vi "File.Folder, Move or Copy.vi"(8 "error in (no error)":errorcluster, 9 "Action":enum16{"Move", "Copy"}(ring), 10 "Dest":path, 11 "Source":path) -> (0 "error out":errorcluster, 3 "Dest Dup":path)   [LabVIEW 2024]
uses:
  Errors/Error.Error Code List.ctl
  <vilib>/KATE/Files/File Utils.lvlib
  Errors.lvlib
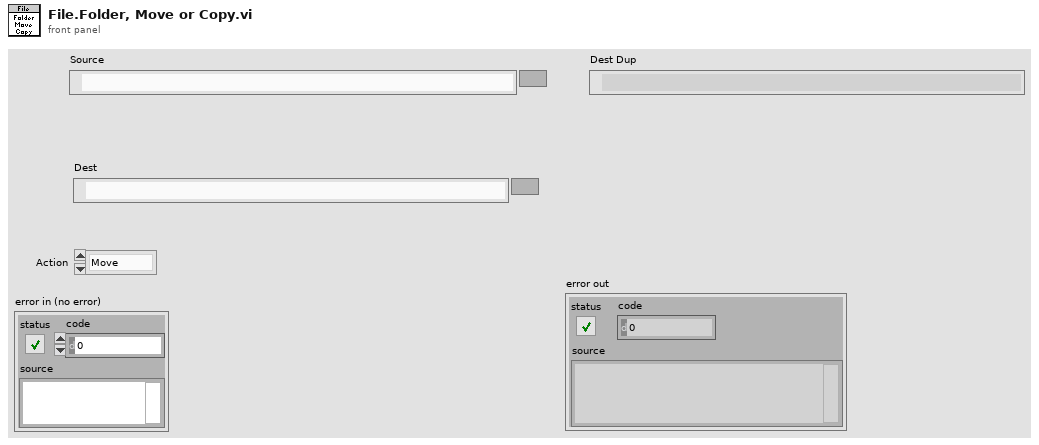
[diagram p1: front panel]
types:
  T1 = typedef "EQMF.lvlib/Errors.lvlib/Error.Error Code List.ctl" = i32
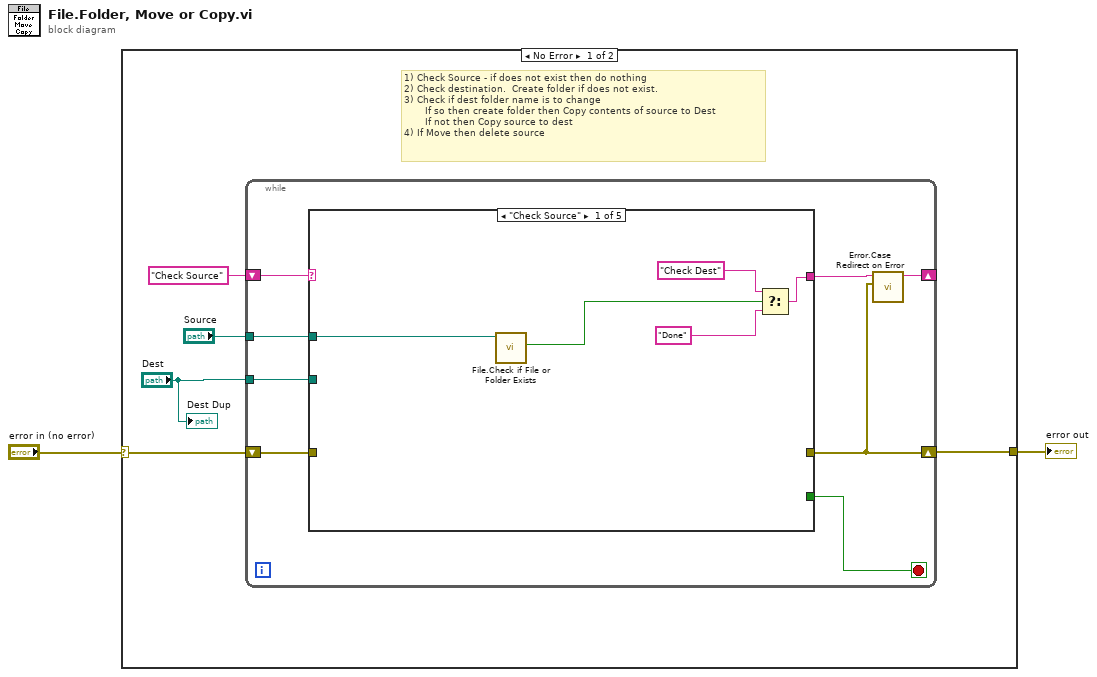
[diagram p0: block diagram]
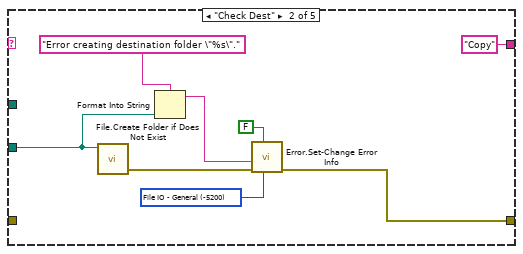
[diagram p2: hidden frame]
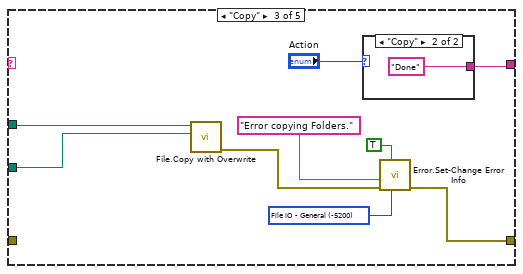
[diagram p3: hidden frame]
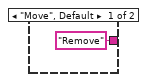
[diagram p4: hidden frame]
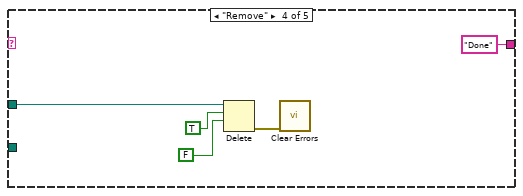
[diagram p5: hidden frame]
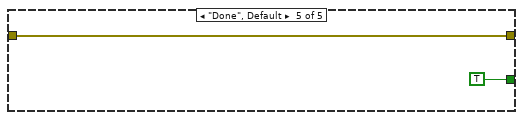
[diagram p6: hidden frame]
diagram:
  n1 = case shown="No Error" "error in (no error)" {
    selector: "error in (no error)" -> [w5 w47]
    tunnel: [w3 w47] -> w1
    frame No Error {
      # "1) Check Source - if does not exist then do nothing\n2) Check destination.  Create folder if does not exist.\n3) Check if dest folder name is to change\n       If so then create folder then Copy contents of source to Dest\n       If not then Copy source to dest\n4) If Move then delete source"
      n2 = while {
        shift-right: [w14] -> _
        shift-left: "Check Source" -> [w15]
        tunnel: "Source" -> [w12]
        tunnel: "Dest" -> [w11]
        shift-right: [w9] -> w3
        shift-left: w5 -> [w10]
        stop <- w8 stop-if-true
        n3 = case shown="\"Check Source\"" w15 {
          tunnel: [w19 "Copy" w36 "Done" _] -> w13
          tunnel: w12 -> [w17 _ w35 w43 _]
          tunnel: w11 -> [_ w25 w34 _ _]
          tunnel: w10 -> [_ _ _ _ w46]
          tunnel: [_ w22 w29 _ w46] -> w9
          tunnel: [_ _ _ _ TRUE] -> w8
          frame "Check Source" {
            n4 = call <vilib>:"File.Check if File or Folder Exists.vi"("Path"=w17) -> ("Exists"=w16:bool)  [unwired: 6 in, 4 out]
            n5 = Select(t="Check Dest", s=w16, f="Done") -> (s? t:f=w19:string)
          }
          frame "Check Dest" {
            w23 = T1 -5200 items=["No Error"=0, "Abort"=-2, "Misc"=-5000, "Fixture Error"=-5100, "File IO - General"=-5200, "FIle IO - Config Error"=-5201, "Instrument - General"=-5300, "Instrument - Serial Com"=-5301, "Instrument - Camera"=-5302, "Instrument - PS"=-5303, "Instrument - Oscilloscope"=-5304, "Instrument - Function Gen"=-5305, "Instrument - Load"=-5306, "Instrument - Meter"=-5307, "Instrument - Power Control"=-5308, "Instrument - Motion"=-5309, "Instrument - RF"=-5310, "System Exe"=-5400, "Image Processing"=-5500, "Communication"=-5600, "Script - Syntax Error"=-6000, "Script - Invalid Name or Param"=-6100, "Script - Timeout"=-6200, "Invalid Data"=-6300, "FW Update Error"=-6500] ("Std Code")
            n6 = call <vilib>:"File.Create Folder if Does Not Exist.vi"("Path"=w25) -> ("error out"=w28:errorcluster)  [unwired: 8 in, 2 out]
            n7 = Format Into String(format string="Error creating destination folder \"%s\".", w25) -> (resulting string=w24:string)  [unwired: 2 in, 1 out]
            n8 = call "Error.Set-Change Error Info.vi"("Std Code"=w23, "Append Details"=FALSE, "error in"=w28, "Description"=w24) -> ("error out"=w22:errorcluster)  [unwired: 7 in]
          }
          frame "Copy" {
            w32 = T1 -5200 items=["No Error"=0, "Abort"=-2, "Misc"=-5000, "Fixture Error"=-5100, "File IO - General"=-5200, "FIle IO - Config Error"=-5201, "Instrument - General"=-5300, "Instrument - Serial Com"=-5301, "Instrument - Camera"=-5302, "Instrument - PS"=-5303, "Instrument - Oscilloscope"=-5304, "Instrument - Function Gen"=-5305, "Instrument - Load"=-5306, "Instrument - Meter"=-5307, "Instrument - Power Control"=-5308, "Instrument - Motion"=-5309, "Instrument - RF"=-5310, "System Exe"=-5400, "Image Processing"=-5500, "Communication"=-5600, "Script - Syntax Error"=-6000, "Script - Invalid Name or Param"=-6100, "Script - Timeout"=-6200, "Invalid Data"=-6300, "FW Update Error"=-6500] ("Std Code")
            n9 = call <vilib>:"File.Copy with Overwrite.vi"("Destination"=w34, "Source"=w35) -> ("error out"=w31:errorcluster)  [unwired: 7 in, 2 out]
            n10 = case shown="\"Copy\"" "Action" {
              tunnel: ["Remove" "Done"] -> w36
              frame "Move", Default {
              }
              frame "Copy" {
              }
            }
            n11 = call "Error.Set-Change Error Info.vi"("Std Code"=w32, "Append Details"=TRUE, "error in"=w31, "Description"="Error copying Folders.") -> ("error out"=w29:errorcluster)  [unwired: 7 in]
          }
          frame "Remove" {
            n12 = Delete(path (use dialog)=w43, entire hierarchy (F)=TRUE, confirm (F)=FALSE) -> (error out=w40:errorcluster)  [unwired: 2 in, 2 out]
            n13 = call <vilib>:"Clear Errors.vi"("error in (no error)"=w40) -> ()  [unwired: 5 in, 2 out]
          }
          frame "Done", Default {
          }
        }
        n14 = call "Error.Case Redirect on Error.vi"("error in"=w9, "Next Case"=w13) -> ("Next Case Out"=w14:string)  [unwired: 9 in]
      }
      "Dest Dup" <- "Dest"
    }
    frame Error {
    }
  }
  "error out" <- w1
